vi "fcs校验 .vi"(1 "string":string) -> (0 "frame check sum":string)   [LabVIEW 2014]
doc: "The Basic Serial Read and Write example performs a Serial Port Read, a Serial Port Write, or a combination of these actions. The user selects the actions (read or write) on the front panel. If both are selected, the VI will write the data first, read data, and then close the VISA session that is opened to the port. This VI will wait until the specified number of bytes is received at the port. Only the number of bytes specified will be read.\n\nINSTRUCTIONS:\n1) Select the serial resource and configuration parameters (baud rate, data bits, parity, stop bits, flow control).\n2) Select the operations to be performed. \n3) Connect the serial port to your device. If no device is available, perform a loopback test by doing one of the following. Short pins 2 and 3 on a RS-232 cable or short pin 4 to pin 8 and pin 5 to pin 9 on a RS-485/422 cable. \n4) Run the VI to see the data read. (The \"read string\" will match the \"string to write\" if a loopback test was performed.)\n\nNote: The parameters set for the serial port must match the parameters of the connected instrument or device. In this example, the bytes to read parameter specifies the number of bytes that the serial port reads. If there were more bytes at the port than the number specified in bytes to read, those bytes would not be read. Also, if you specify to read more bytes than the number of bytes actually read, you might receive a timeout error message.\n\nOn the block diagram, the Configure Serial Port VI sets the configuration parameters. The front panel displays the controls used to configure the basic parameters, such as baud rate, data bits, and parity. Constants configure the other parameters the user probably does not need set. After the VISA Configure Serial Port VI opens the VISA session and configures the port, the VI passes the VISA resource name to other VIs that perform operations on that VISA resource. The VISA Write function sends a command to the serial device and the VISA Read function returns data based on the command. The VISA Close function then closes the reference to the serial device. It is important to close the reference; otherwise communication through with that port through protocols other than VISA might not be possible."
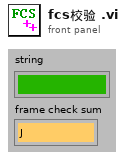
[diagram p1: front panel]
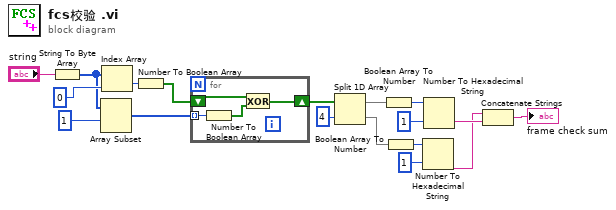
[diagram p0: block diagram]
diagram:
  n1 = String To Byte Array(string="string") -> (unsigned byte array=w4:u8[])
  n2 = Array Subset ("数组子集")(array=w4, index=1) -> (w1:u8[])  [unwired: 1 in]
  n3 = Index Array(array=w4, index=0) -> (element=w2:u8)
  n4 = Number To Boolean Array(number=w2) -> (Boolean array=w3:bool[])
  n5 = for {
    tunnel: w1 -> [w20] mode=indexing
    shift-right: [w22] -> w12
    shift-left: w3 -> [w21]
    n6 = Number To Boolean Array(number=w20) -> (Boolean array=w19:bool[])
    n7 = Exclusive Or(1:w19, 2:w21) -> (0:w22:bool[])
  }
  n8 = Split 1D Array(array=w12, index=4) -> (first subarray=w18:bool[], second subarray=w13:bool[])
  n9 = Boolean Array To Number(Boolean array=w18) -> (number=w14:u32)
  n10 = Boolean Array To Number(Boolean array=w13) -> (number=w15:u32)
  n11 = Number To Hexadecimal String(1:1 ("index"), 2:w15) -> (0:w16:string)
  n12 = Number To Hexadecimal String(1:1 ("index"), 2:w14) -> (0:w17:string)
  n13 = Concatenate Strings(w16, w17) -> (→"frame check sum":string)
